vi "处理8邻域.vi"(0 "图片":picture, 5 "地图":dbl[][](array[numeric]), 7 "雷区":dbl[][](array[numeric]), 9 "行":i16, 11 "列":i16) -> (4 "图片 2":picture, 6 "地图 2":dbl[][](array[numeric]))   [LabVIEW 2023]
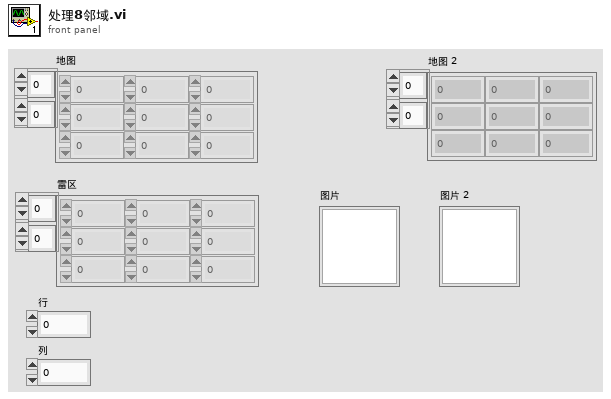
[diagram p1: front panel]
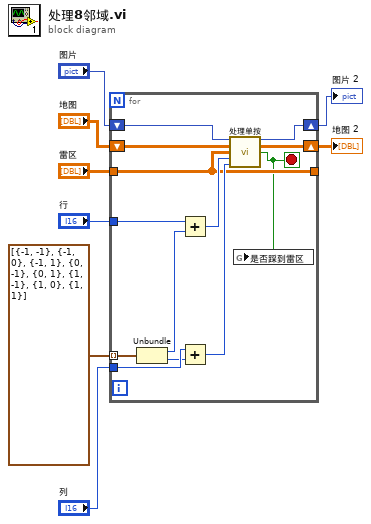
[diagram p0: block diagram]
diagram:
  n1 = for {
    tunnel: cluster{i32, i32}[] [{-1, -1}, {-1, 0}, {-1, 1}, {0, -1}, {0, 1}, {1, -1}, {1, 0}, {1, 1}] -> [w15] mode=indexing
    shift-right: [w19] -> w1
    shift-left: "地图" -> [w16]
    tunnel: "行" -> [w21]
    tunnel: "列" -> [w20]
    shift-right: [w18] -> w2
    shift-left: "图片" -> [w17]
    tunnel: "雷区" -> [w10]
    tunnel: [w10] -> _
    stop <- w9 stop-if-true
    n2 = Unbundle(w15) -> (w14:i32, w13:i32)
    n3 = Add(x=w21, y=w14) -> (x+y=w12:i32)
    n4 = Add(x=w20, y=w13) -> (x+y=w11:i32)
    n5 = call "处理单按.vi"("图片"=w17, "地图"=w16, "雷区"=w10, "行"=w12, "列"=w11) -> ("图片 2"=w18:picture, "地图 2"=w19:dbl[][], "是否踩雷"=w9:bool)  [unwired: 7 in, 1 out]
    n6 = global write "全局变量.vi" "是否踩到雷区"(w9) -> ()
  }
  "地图 2" <- w1
  "图片 2" <- w2
